vi "串口设置.vi"() -> ()   [LabVIEW 2014]
panel:
  in  "返回":bool
  in  "确定":bool
  in  "串口设置":T1={"通讯串口"="COM1", "波特率"=9600, "数据比特"=8, "奇偶校验"=enum."None", "停止位"=10, "等待延时(ms)"=0} {"停止位" items=["1.0"=10, "1.5"=15, "2.0"=20]; "数据比特" min=5 max=8 step=1; "波特率" items=["75"=75, "110"=110, "134"=134, "150"=150, "300"=300, "600"=600, "1200"=1200, "1800"=1800, "2400"=2400, "4800"=4800, "7200"=7200, "9600"=9600, "14400"=14400, "19200"=19200, "28800"=28800, "38400"=38400, "56000"=56000, "57600"=57600, "115200"=115200, "128000"=128000, "230400"=230400]}
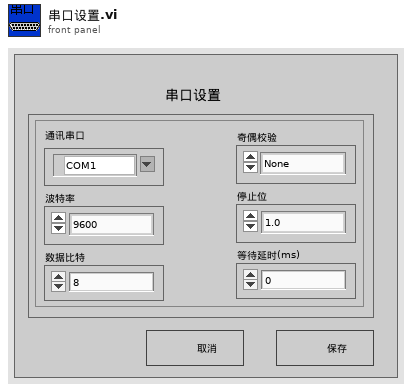
[diagram p1: front panel]
types:
  T1 = cluster{"通讯串口":refnum<visa-resource-name>, "波特率":u32, "数据比特":u16, "奇偶校验":enum16{"None", "Odd", "Even", "Mark", "Space"}, "停止位":u16, "等待延时(ms)":u32}
  T2 = enum16{"open", "replace", "create", "open or create", "replace or create", "replace or create with confirmation"}
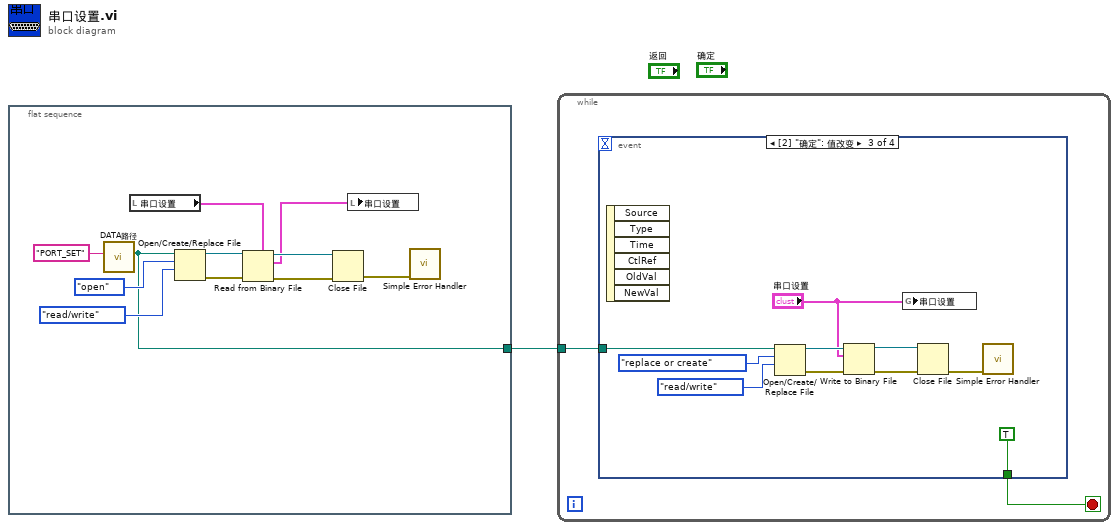
[diagram p0: block diagram]
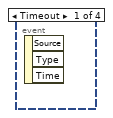
[diagram p2: hidden frame]
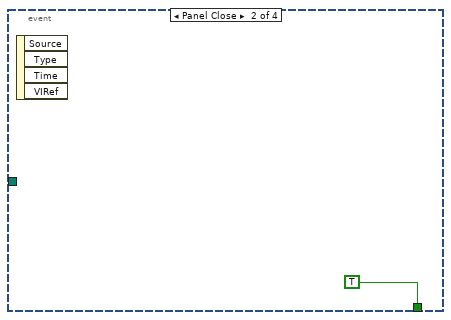
[diagram p3: hidden frame]
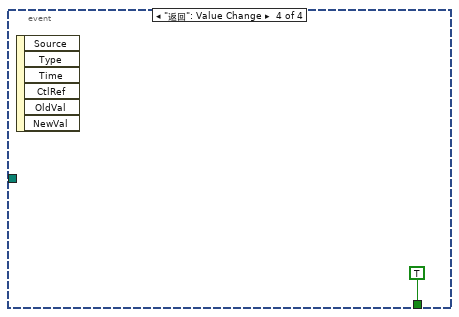
[diagram p4: hidden frame]
diagram:
  n1 = flat-sequence {
    tunnel: [w2] -> w1
    frame #0 {
      n2 = call "DATA路径.vi"("文件名"="PORT_SET") -> ("DATA路径"=w2:path)  [unwired: 10 in]
      n3 = local read "串口设置"() -> (w7:T1)
      n4 = Open/Create/Replace File(file path (use dialog)=w2, operation (0:open)=T2."open" ("操作(0:open)"), access (0:read/write)=enum16{"read/write", "read-only", "write-only"}."read/write" ("权限(0:read/write)")) -> (refnum out=w9:refnum<file>, error out=w8:errorcluster)  [unwired: 3 in, 1 out]
      n5 = Read from Binary File(5:w7, 8:w8, 11:w9) -> (0:w5:errorcluster, 2:w3:T1, 3:w6:refnum<file>)  [unwired: 3 in, 1 out]
      n6 = Close File(refnum=w6, error in=w5) -> (error out=w4:errorcluster)  [unwired: 1 out]
      n7 = local write "串口设置"(w3) -> ()
      n8 = call <vilib>:"Simple Error Handler.vi"("error in (no error)"=w4) -> ()  [unwired: 4 in, 5 out]
    }
  }
  n9 = while {
    tunnel: w1 -> [w14]
    stop <- w13 stop-if-true
    n10 = event shown="[2] \"确定\": 值改变" {
      selector: _ -> [_ _ _ _]
      dyn-events: _ -> [_ _ _ _]
      timeout: _ -> [_ _ _ _]
      tunnel: w14 -> [_ _ w19 _]
      tunnel: [_ TRUE TRUE TRUE] -> w13
      event Timeout {
        n11 = event-data() -> ()  [unwired: 1 in, 3 out]
      }
      event Panel Close {
        n12 = event-data() -> ()  [unwired: 1 in, 4 out]
      }
      event "确定": Value Change {
        n13 = event-data() -> ()  [unwired: 1 in, 6 out]
        n14 = Open/Create/Replace File(file path (use dialog)=w19, operation (0:open)=T2."replace or create" ("操作(0:open)"), access (0:read/write)=enum16{"read/write", "read-only", "write-only"}."read/write" ("权限(0:read/write)")) -> (refnum out=w23:refnum<file>, error out=w24:errorcluster)  [unwired: 3 in, 1 out]
        n15 = Write to Binary File(file (use dialog)=w23, data="串口设置", error in=w24) -> (refnum out=w21:refnum<file>, error out=w22:errorcluster)  [unwired: 3 in, 1 out]
        n16 = global write "三菱全局变量.vi" "串口设置"("串口设置") -> ()
        n17 = Close File(refnum=w21, error in=w22) -> (error out=w20:errorcluster)  [unwired: 1 out]
        n18 = call <vilib>:"Simple Error Handler.vi"("error in (no error)"=w20) -> ()  [unwired: 4 in, 5 out]
      }
      event "返回": Value Change {
        n19 = event-data() -> ()  [unwired: 1 in, 6 out]
      }
    }
  }
